vi "Main Process Case.vi"(8 "error in (no error)":errorcluster, 10 "CurrentAction":string, 11 "MPC_Laser Marked in":refnum<class "MPC_Laser Marked.lvclass">) -> (0 "error out":errorcluster, 1 "keepCase":bool, 3 "MPC_Laser Marked out":refnum<class "MPC_Laser Marked.lvclass">)   [LabVIEW 2019, in "MPC_Laser Marked.lvclass"]
uses:
  MPC_Laser Marked.lvclass
  Function/IO Folder/IO_VI/IOCtrl/Ctrl/DMC1000B_1 SelectIn.ctl
  Function/IO Folder/IO_VI/IOCtrl/Ctrl/DMC1000B_1 SelectOutput.ctl
  Function/Main UI/Ctrl/XY Table Action.ctl
  Function/UpVision/Ctrl/UpColorImg.ctl
  Function/UpVision/Ctrl/UpEnum_VisionCalibSet_Act.ctl
  Function/UpVision/Ctrl/UpGrayImg.ctl
  Function/Axis/Axis_Class/SubVI/Axis Motion/Axis_Go Point.vi
  Function/Main UI/Glb/Main_UI Gb.vi
  LLB/Commonly VI/Main Glb.vi
  LLB/Commonly VI.lvlib
  LLB/Message/MsgShowAndLog.lvlib
panel:
  out "Current Index":i32
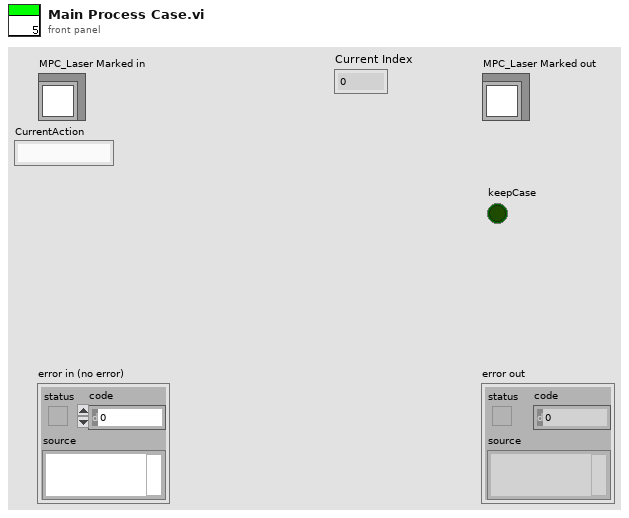
[diagram p1: front panel]
types:
  T1 = cluster{"AutoRunFlg":refnum<vi>, "Action Finish Flg":refnum<vi>, "Remaining Action":refnum<vi>, "Btn_AutoRun":refnum<vi>, "Manual Flg":refnum<vi>, "Sub Process Error":refnum<vi>}
  T2 = typedef "DMC1000B_1 SelectIn.ctl" = enum16{"M_IN00預備", "M_IN01緊急急停檢測", "M_IN02啟動按鈕綠色", "M_IN03正壓氣壓檢知", "M_IN04安全門感知", "M_IN05接受前機台有料#1信號", "M_IN06接受前機台有料#2信號", "M_IN07接受後機台要料#3信號", "M_IN08接受後機台要料#4信號", "M_IN09軌道載板前進料到位檢知", "M_IN10到料阻擋氣缸上位檢知(阻擋位)", "M_IN11到料阻擋氣缸下位檢知(阻擋位)", "M_IN12上頂固定載板氣缸上位檢知", "M_IN13上頂固定載板氣缸下位檢知", "M_IN14軌道載板到位減速檢知", "M_IN15軌道載板到位檢知", "M_IN16軌道載板後出料檢知", "M_IN17", "M_IN18", "M_IN19", "M_IN20", "M_IN21第一軸準備輸入信號 RDY", "M_IN22第二軸準備輸入信號 RDY", "M_IN23第三軸準備輸入信號 RDY", "M_IN24", "M_IN25第一軸ALM+(  伺服警報輸出  )", "M_IN26第二軸ALM+(  伺服警報輸出  )", "M_IN27第三軸ALM+(  伺服警報輸出  )", "M_IN28", "M_IN29第一軸定位完成信號 INP", "M_IN30第二軸定位完成信號 INP", "M_IN31第三軸定位完成信號 INP", "M_IN32"}
  T3 = typedef "DMC1000B_1 SelectOutput.ctl" = enum16{"M_Out0預備", "M_OUT01蜂鳴器", "M_OUT02紅燈", "M_OUT03綠燈", "M_OUT04黃燈", "M_OUT05上頂固定位氣缸電磁閥", "M_OUT06到料阻擋氣缸電磁閥", "M_OUT07向前機台發出要料#1信號", "M_OUT08向前機台發出要料#2信號", "M_OUT09向後機台發出有料#3信號", "M_OUT10向後機台發出有料#4信號", "M_OUT11接駁台馬達啟動開/關", "M_OUT12接駁台馬達慢速", "M_OUT13抽風機開/關", "M_OUT14上視覺上光源", "M_OUT15DC吹風扇開/關", "M_OUT16Z軸煞車釋放", "M_OUT17", "M_OUT18", "M_OUT19", "M_OUT20", "M_OUT21", "M_OUT22", "M_OUT23", "M_OUT24", "M_OUT25第一軸SEVON1伺服使能信號", "M_OUT26第二軸SEVON2伺服使能信號", "M_OUT27第三軸SEVON3伺服使能信號"}
  T4 = typedef "XY Table Action.ctl" = enum16{"Check Mark", "Check Z", "Laser", "Request Action"}
  T5 = enum16{"Initial", "Load", "Save", "Read", "WriteSpeed", "WritePoint"}
  T6 = cluster{"index":i32, "Mark 1Vision":cluster{"Position":cluster{"x":sgl, "y":sgl}, "Angle":sgl, "Score":sgl}, "OK/NG":bool}
  T7 = typedef "UpEnum_VisionCalibSet_Act.ctl" = enum16{"initial", "initialref", "save", "load", "UpDataToUI", "write", "read"}
  T8 = typedef "UpColorImg.ctl" = enum16{"CUpCam", "CUpSource", "CUpShow", "CUpToProcess1", "CUpToProcess2", "CUpForMatch", "CUpForCheckNumbers", "CupPreProcess"}
  T9 = typedef "UpGrayImg.ctl" = enum16{"CUpGray", "CUpProce1", "CUpProce2", "UpPattern1", "UpPattern2", "UpCalibImg", "UpPreProcess"}
  T10 = typedef "IMAQ Image.ctl" = refnum<image>
  T11 = cluster{"Position":cluster{"x":sgl, "y":sgl}, "Angle":sgl, "Score":sgl}
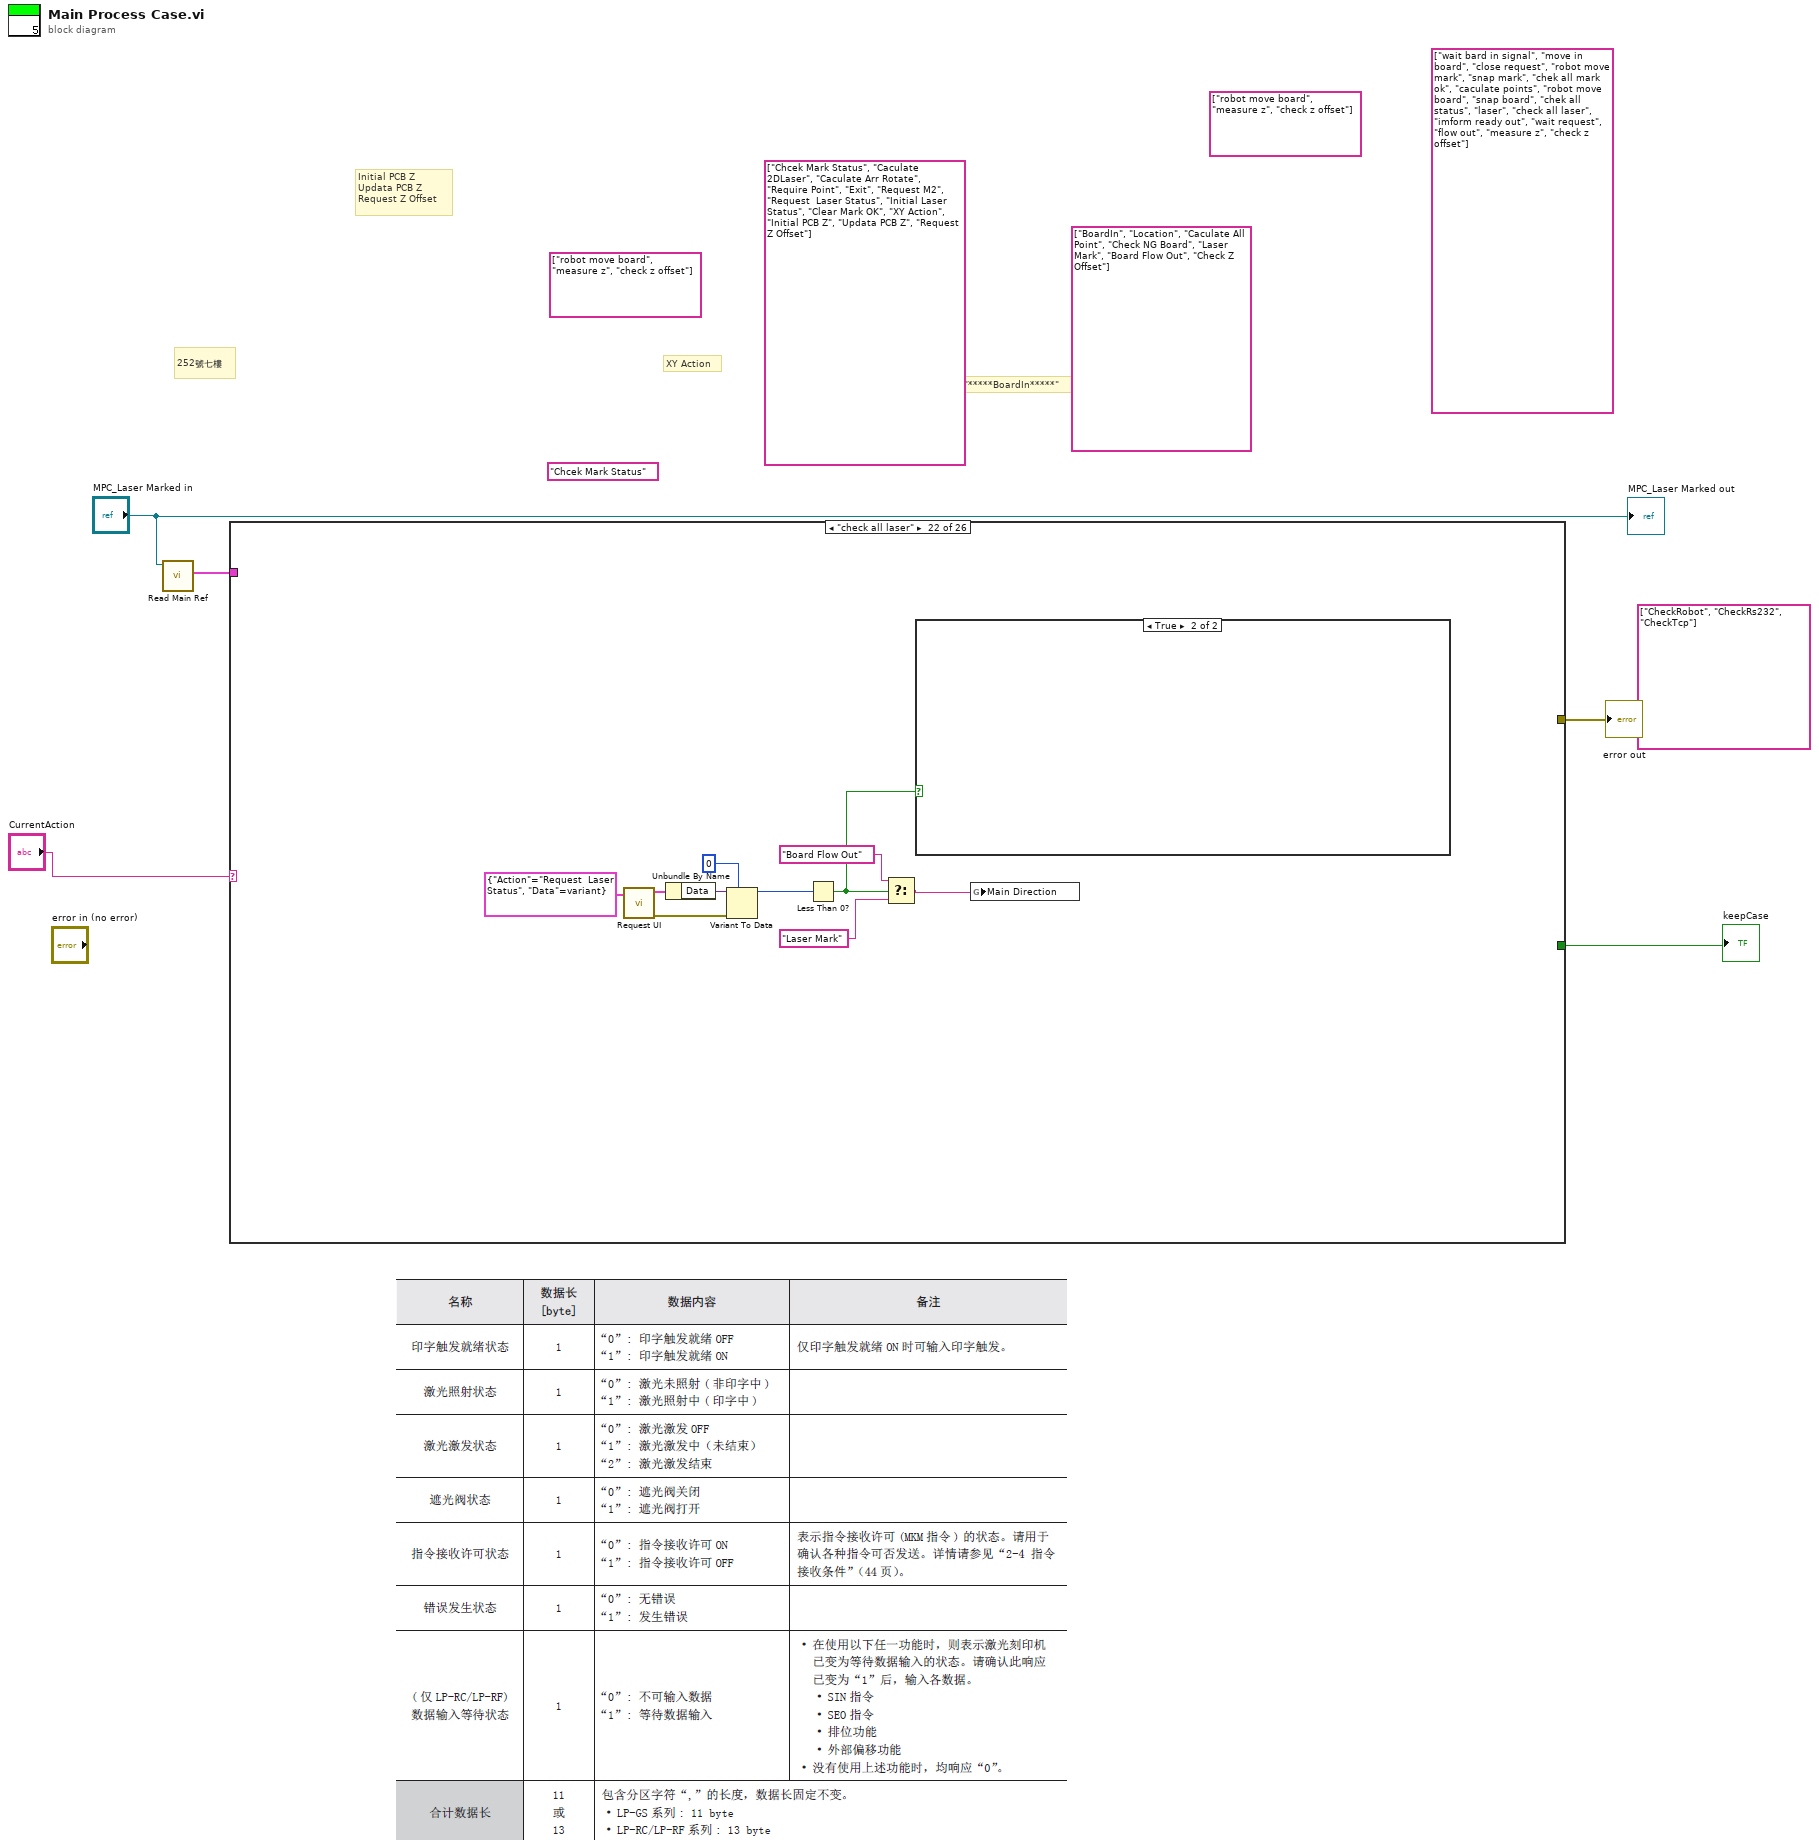
[diagram p0: block diagram]
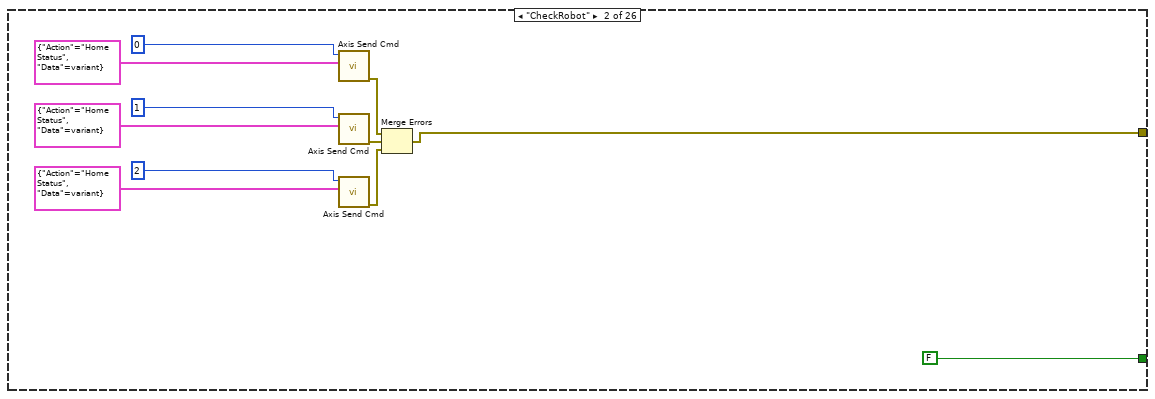
[diagram p3: hidden frame]
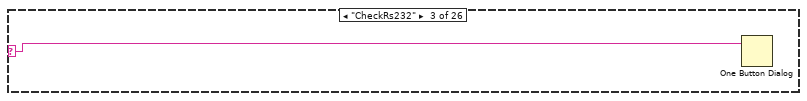
[diagram p4: hidden frame]
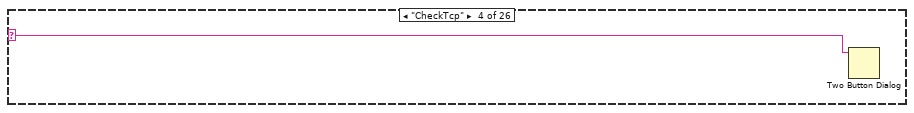
[diagram p5: hidden frame]
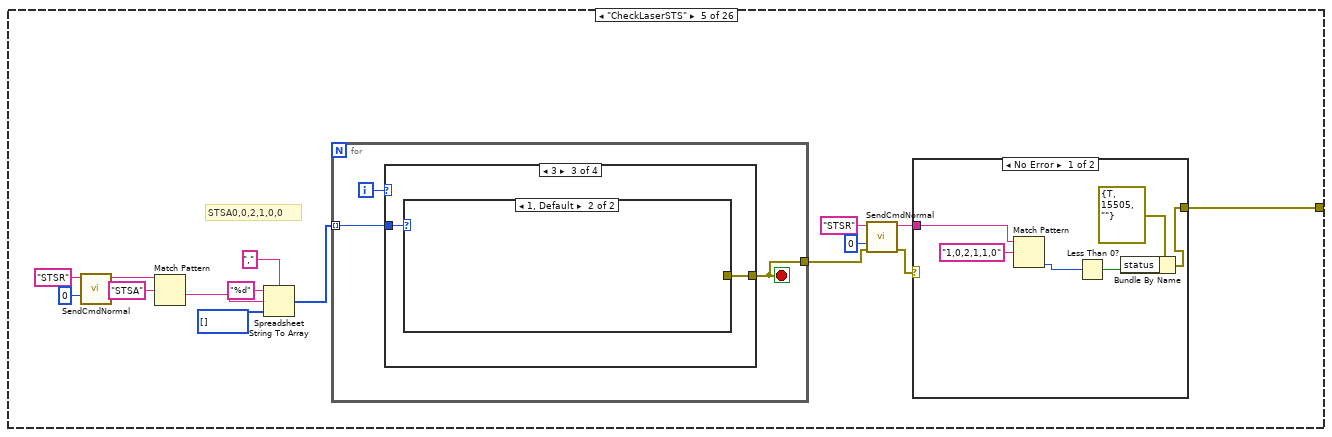
[diagram p6: hidden frame]
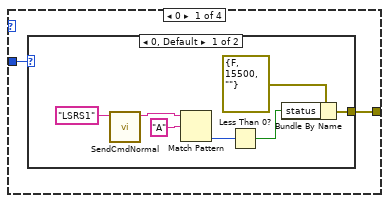
[diagram p8: hidden frame]
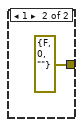
[diagram p9: hidden frame]
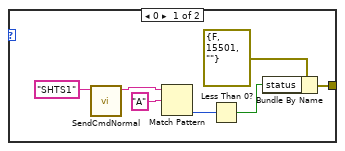
[diagram p12: hidden frame]
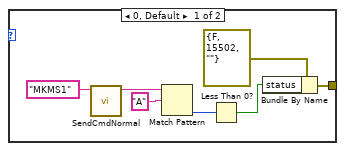
[diagram p14: hidden frame]
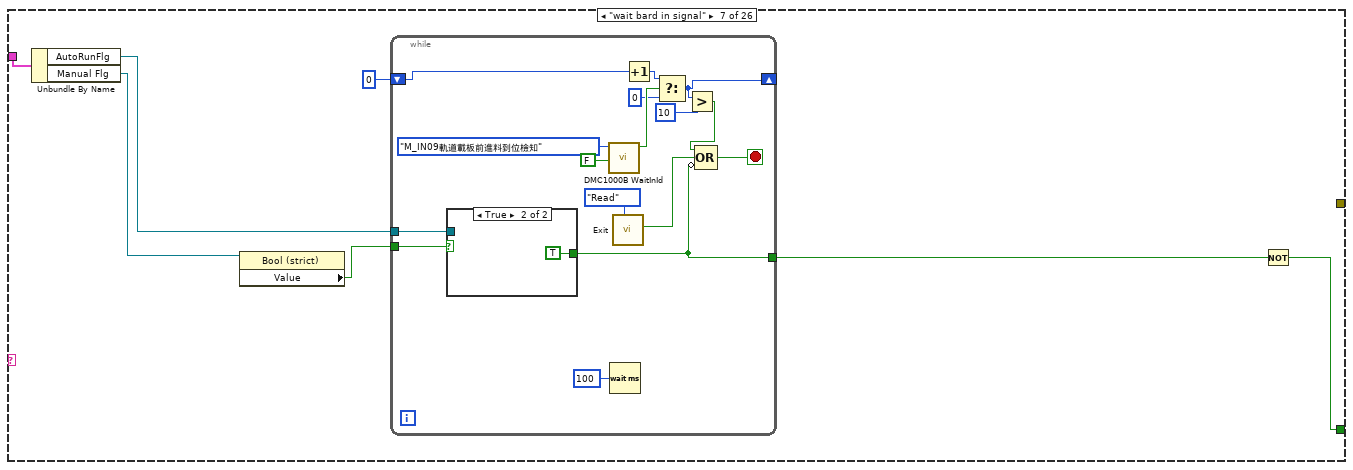
[diagram p16: hidden frame]
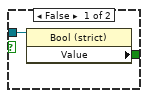
[diagram p17: hidden frame]
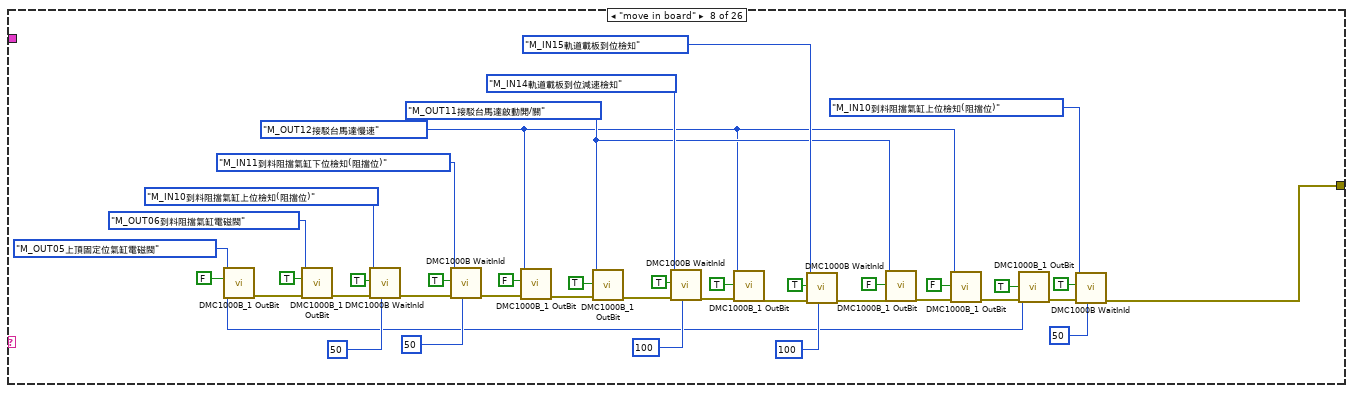
[diagram p18: hidden frame]
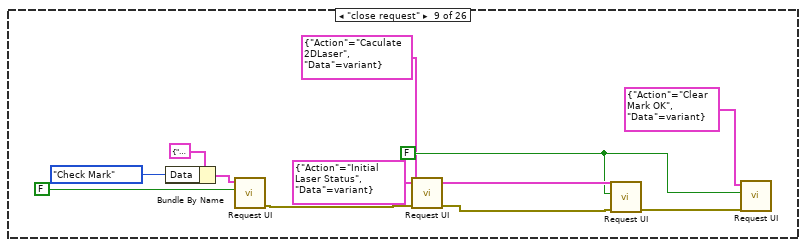
[diagram p19: hidden frame]
diagram:
  (unwired) "Chcek Mark Status" ("Action")
  (unwired) string[] ["robot move board", "measure z", "check z offset"]
  (unwired) string[] ["Chcek Mark Status", "Caculate 2DLaser", "Caculate Arr Rotate", "Require Point", "Exit", "Request M2", "Request  Laser Status", "Initial Laser Status", "Clear Mark OK", "XY Action", "Initial PCB Z", "Updata PCB Z", "Request Z Offset"]
  (unwired) string[] ["robot move board", "measure z", "check z offset"]
  (unwired) string[] ["wait bard in signal", "move in board", "close request", "robot move mark", "snap mark", "chek all mark ok", "caculate points", "robot move board", "snap board", "chek all status", "laser", "check all laser", "imform ready out", "wait request", "flow out", "measure z", "check z offset"]
  (unwired) string[] ["BoardIn", "Location", "Caculate All Point", "Check NG Board", "Laser Mark", "Board Flow Out", "Check Z Offset"]
  (unwired) string[] ["CheckRobot", "CheckRs232", "CheckTcp"] ("Process")
  # "252號七樓"
  # "Initial PCB Z\nUpdata PCB Z\nRequest Z Offset"
  # "XY Action"
  # "\"*****BoardIn*****\""
  n1 = call-dynamic "Read Main Ref.vi"("Main Process Class in"="MPC_Laser Marked in") -> ("Main Ref"=w2:T1)  [unwired: 8 in, 2 out]
  n2 = case shown="\"check all laser\"" "CurrentAction" {
    selector: "CurrentAction" -> [_ _ w17 w18 _ _ _ _ _ _ _ _ _ _ _ _ _ _ _ _ _ _ _ _ _ _]
    tunnel: [_ FALSE _ _ _ _ w77 _ _ _ _ _ _ _ _ _ _ _ _ _ _ _ _ w379 _ _] -> w4
    tunnel: w2 -> [_ _ _ _ _ _ w79 _ _ _ _ _ _ _ _ _ _ _ _ _ _ _ _ w382 _ _]
    tunnel: [_ w6 _ _ w19 _ _ w99 _ _ w156 w190 _ _ _ _ w260 w325 _ _ w356 _ _ _ w403 w410] -> w1
    frame Default {
    }
    frame "CheckRobot" {
      n3 = call "Axis Send Cmd.vi"("DataIn"=cluster{"Action":string, "Data":variant} {"Action"="Home Status", "Data"=variant}, "Axis Index"=0) -> ("Error Out"=w9:errorcluster)  [unwired: 9 in]
      n4 = call "Axis Send Cmd.vi"("DataIn"=cluster{"Action":string, "Data":variant} {"Action"="Home Status", "Data"=variant}, "Axis Index"=1) -> ("Error Out"=w8:errorcluster)  [unwired: 9 in]
      n5 = call "Axis Send Cmd.vi"("DataIn"=cluster{"Action":string, "Data":variant} {"Action"="Home Status", "Data"=variant}, "Axis Index"=2) -> ("Error Out"=w7:errorcluster)  [unwired: 9 in]
      n6 = Merge Errors(w9, w8, w7) -> (w6:errorcluster)
    }
    frame "CheckRs232" {
      n7 = One Button Dialog(message=w17) -> ()  [unwired: 1 in, 1 out]
    }
    frame "CheckTcp" {
      n8 = Two Button Dialog(message=w18) -> ()  [unwired: 2 in, 1 out]
    }
    frame "CheckLaserSTS" {
      # "STSA0,0,2,1,0,0"
      n9 = call "SendCmdNormal.vi"("index"=0, "DataIn"="STSR") -> ("Reccmd"=w31:string)  [unwired: 7 in, 2 out]
      n10 = Match Pattern(string=w31, regular expression="STSA") -> (after substring=w29:string)  [unwired: 1 in, 3 out]
      n11 = Spreadsheet String To Array(delimiter (Tab)=",", format string="%d", spreadsheet string=w29, array type (2D Dbl)=i32[] []) -> (array=w25:i32[])
      n12 = for {
        tunnel: w25 -> [w43] mode=indexing
        tunnel: [w41] -> w22
        i -> [w42]
        stop <- w41 stop-if-true
        n13 = case shown="3" w42 {
          tunnel: w43 -> [w45 w54 w56 w65]
          tunnel: [w44 _ w55 w64] -> w41
          frame 0 {
            n14 = case shown="0, Default" w45 {
              tunnel: [w47 errorcluster {"status"=FALSE, "code"=0, "source"=""} ("error out")] -> w44
              frame 0, Default {
                n15 = call "SendCmdNormal.vi"("DataIn"="LSRS1") -> ("Reccmd"=w51:string)  [unwired: 8 in, 2 out]
                n16 = Match Pattern(string=w51, regular expression="A") -> (offset past match=w49:i32)  [unwired: 1 in, 3 out]
                n17 = Less Than 0?(x=w49) -> (x < 0?=w46:bool)
                n18 = Bundle By Name(cluster=errorcluster {"status"=FALSE, "code"=15500, "source"=""} ("error constant"), "status"=w46) -> (w47:errorcluster)
              }
              frame 1 {
              }
            }
          }
          frame 1, Default {
            n19 = case shown="0, Default" w54 {
              frame 0, Default {
              }
              frame 1 {
              }
            }
          }
          frame 3 {
            n20 = case shown="1, Default" w56 {
              tunnel: [w57 _] -> w55
              frame 0 {
                n21 = call "SendCmdNormal.vi"("DataIn"="SHTS1") -> ("Reccmd"=w63:string)  [unwired: 8 in, 2 out]
                n22 = Match Pattern(string=w63, regular expression="A") -> (offset past match=w62:i32)  [unwired: 1 in, 3 out]
                n23 = Less Than 0?(x=w62) -> (x < 0?=w61:bool)
                n24 = Bundle By Name(cluster=errorcluster {"status"=FALSE, "code"=15501, "source"=""} ("error constant"), "status"=w61) -> (w57:errorcluster)
              }
              frame 1, Default {
              }
            }
          }
          frame 4 {
            n25 = case shown="1" w65 {
              tunnel: [w66 _] -> w64
              frame 0, Default {
                n26 = call "SendCmdNormal.vi"("DataIn"="MKMS1") -> ("Reccmd"=w72:string)  [unwired: 8 in, 2 out]
                n27 = Match Pattern(string=w72, regular expression="A") -> (offset past match=w71:i32)  [unwired: 1 in, 3 out]
                n28 = Less Than 0?(x=w71) -> (x < 0?=w70:bool)
                n29 = Bundle By Name(cluster=errorcluster {"status"=FALSE, "code"=15502, "source"=""} ("error constant"), "status"=w70) -> (w66:errorcluster)
              }
              frame 1 {
              }
            }
          }
        }
      }
      n30 = call "SendCmdNormal.vi"("error in (no error)"=w22, "index"=0, "DataIn"="STSR") -> ("error out"=w21:errorcluster, "Reccmd"=w20:string)  [unwired: 6 in, 1 out]
      n31 = case shown="No Error" w21 {
        selector: w21 -> [_ w40]
        tunnel: w20 -> [w39 _]
        tunnel: [w34 w40] -> w19
        frame No Error {
          n32 = Match Pattern(string=w39, regular expression="1,0,2,1,1,0") -> (offset past match=w37:i32)  [unwired: 1 in, 3 out]
          n33 = Less Than 0?(x=w37) -> (x < 0?=w36:bool)
          n34 = Bundle By Name(cluster=errorcluster {"status"=TRUE, "code"=15505, "source"=""} ("error constant"), "status"=w36) -> (w34:errorcluster)
        }
        frame Error {
        }
      }
    }
    frame "*****BoardIn*****" {
    }
    frame "wait bard in signal" {
      n35 = Unbundle By Name(w79) -> ("AutoRunFlg"=w75:refnum<vi>, "Manual Flg"=w74:refnum<vi>)
      n36 = property class="Bool (strict)"(reference=w74) -> ("Value"=w73:bool)  [unwired: 1 in, 2 out]
      n37 = while {
        tunnel: w75 -> [w92]
        tunnel: [w89] -> w78
        shift-right: [w83] -> _
        shift-left: 0 -> [w85]
        tunnel: w73 -> [w80]
        stop <- w90 stop-if-true
        n38 = case shown="True" w80 {
          tunnel: w92 -> [w97 _]
          tunnel: [w96 TRUE ("Value")] -> w89
          frame False {
            n39 = property class="Bool (strict)"(reference=w97) -> ("Value"=w96:bool)  [unwired: 1 in, 2 out]
          }
          frame True {
          }
        }
        n40 = call "DMC1000B WaitInId.vi"("Wait?"=FALSE, "64IIN_4 Select"=DMC1000B_1_SelectIn."M_IN09軌道載板前進料到位檢知") -> ("StatusOut"=w87:bool)  [unwired: 7 in, 2 out]
        n41 = Wait (ms)(milliseconds to wait=u32 100) -> ()  [unwired: 1 out]
        n42 = call "Exit.vi"("Enum"=enum16{"Initial", "Read", "Write"}."Read") -> ("ExitOut"=w91:bool)  [unwired: 10 in]
        n43 = Increment(x=w85) -> (x+1=w86:i32)
        n44 = Select(t=w86, s=w87, f=0) -> (s? t:f=w83:i32)
        n45 = Greater?(x=w83, y=10) -> (0:w81:bool)
        n46 = Compound Arithmetic op=OR(w81, w91, invert w89) -> (w90:bool)
      }
      n47 = Not(x=w78) -> (.not. x?=w77:bool)
    }
    frame "move in board" {
      w107 = DMC1000B_1_SelectOutput."M_OUT12接駁台馬達慢速" ("IO_Output_1 Select")
      w110 = DMC1000B_1_SelectOutput."M_OUT11接駁台馬達啟動開/關" ("IO_Output_1 Select")
      w104 = DMC1000B_1_SelectOutput."M_OUT05上頂固定位氣缸電磁閥" ("IO_Output_1 Select")
      n48 = call "DMC1000B_1 OutBit.vi"("BL"=FALSE, "IO_Output_1 Select"=w104) -> ("error out"=w128:errorcluster)  [unwired: 9 in]
      n49 = call "DMC1000B_1 OutBit.vi"("error in (no error)"=w128, "BL"=TRUE, "IO_Output_1 Select"=DMC1000B_1_SelectOutput."M_OUT06到料阻擋氣缸電磁閥") -> ("error out"=w133:errorcluster)  [unwired: 8 in]
      n50 = call "DMC1000B WaitInId.vi"("time(0.1)"=50, "error in"=w133, "Status"=TRUE, "64IIN_4 Select"=DMC1000B_1_SelectIn."M_IN10到料阻擋氣缸上位檢知(阻擋位)") -> ("error Out"=w127:errorcluster)  [unwired: 5 in, 2 out]
      n51 = call "DMC1000B WaitInId.vi"("time(0.1)"=50, "error in"=w127, "Status"=TRUE, "64IIN_4 Select"=DMC1000B_1_SelectIn."M_IN11到料阻擋氣缸下位檢知(阻擋位)") -> ("error Out"=w116:errorcluster)  [unwired: 5 in, 2 out]
      n52 = call "DMC1000B_1 OutBit.vi"("error in (no error)"=w116, "BL"=FALSE, "IO_Output_1 Select"=w107) -> ("error out"=w115:errorcluster)  [unwired: 8 in]
      n53 = call "DMC1000B_1 OutBit.vi"("error in (no error)"=w115, "BL"=TRUE, "IO_Output_1 Select"=w110) -> ("error out"=w124:errorcluster)  [unwired: 8 in]
      n54 = call "DMC1000B WaitInId.vi"("time(0.1)"=100, "error in"=w124, "Status"=TRUE, "64IIN_4 Select"=DMC1000B_1_SelectIn."M_IN14軌道載板到位減速檢知") -> ("error Out"=w118:errorcluster)  [unwired: 5 in, 2 out]
      n55 = call "DMC1000B_1 OutBit.vi"("error in (no error)"=w118, "BL"=TRUE, "IO_Output_1 Select"=w107) -> ("error out"=w117:errorcluster)  [unwired: 8 in]
      n56 = call "DMC1000B WaitInId.vi"("time(0.1)"=100, "error in"=w117, "Status"=TRUE, "64IIN_4 Select"=DMC1000B_1_SelectIn."M_IN15軌道載板到位檢知") -> ("error Out"=w111:errorcluster)  [unwired: 5 in, 2 out]
      n57 = call "DMC1000B_1 OutBit.vi"("error in (no error)"=w111, "BL"=FALSE, "IO_Output_1 Select"=w110) -> ("error out"=w108:errorcluster)  [unwired: 8 in]
      n58 = call "DMC1000B_1 OutBit.vi"("error in (no error)"=w108, "BL"=FALSE, "IO_Output_1 Select"=w107) -> ("error out"=w105:errorcluster)  [unwired: 8 in]
      n59 = call "DMC1000B_1 OutBit.vi"("error in (no error)"=w105, "BL"=TRUE, "IO_Output_1 Select"=w104) -> ("error out"=w103:errorcluster)  [unwired: 8 in]
      n60 = call "DMC1000B WaitInId.vi"("time(0.1)"=50, "error in"=w103, "Status"=TRUE, "64IIN_4 Select"=DMC1000B_1_SelectIn."M_IN10到料阻擋氣缸上位檢知(阻擋位)") -> ("error Out"=w99:errorcluster)  [unwired: 5 in, 2 out]
    }
    frame "close request" {
      w146 = FALSE ("Wait Reply")
      n61 = Bundle By Name(cluster=cluster{"Action":string, "Data":variant} {"Action"="XY Action", "Data"=variant} ("Data"), "Data"=XY_Table_Action."Check Mark" ("XY Table Action")) -> (w143:cluster{"Action":string, "Data":variant})
      n62 = call "Request UI.vi"("Wait Reply"=FALSE, "Data"=w143) -> ("error out"=w141:errorcluster)  [unwired: 8 in, 1 out]
      n63 = call "Request UI.vi"("error in (no error)"=w141, "Data"=cluster{"Action":string, "Data":variant} {"Action"="Caculate 2DLaser", "Data"=variant}) -> ("error out"=w144:errorcluster)  [unwired: 8 in, 1 out]
      n64 = call "Request UI.vi"("error in (no error)"=w144, "Wait Reply"=w146, "Data"=cluster{"Action":string, "Data":variant} {"Action"="Initial Laser Status", "Data"=variant}) -> ("error out"=w147:errorcluster)  [unwired: 7 in, 1 out]
      n65 = call "Request UI.vi"("error in (no error)"=w147, "Wait Reply"=w146, "Data"=cluster{"Action":string, "Data":variant} {"Action"="Clear Mark OK", "Data"=variant}) -> ()  [unwired: 7 in, 2 out]
    }
    frame "*****Location*****" {
    }
    frame "robot move mark" {
      n66 = call "Request UI.vi"("Data"=cluster{"Action":string, "Data":variant} {"Action"="Chcek Mark Status", "Data"=variant}) -> ("DataOut"=w154:cluster{"Action":string, "Data":variant})  [unwired: 9 in, 1 out]
      n67 = Unbundle By Name(w154) -> ("Data"=w153:variant)
      n68 = Variant To Data(type=cluster{"M1":bool, "M2":bool} {"M1"=TRUE, "M2"=TRUE}, Variant=w153) -> (data=w151:cluster{"M1":bool, "M2":bool})  [unwired: 1 in, 1 out]
      n69 = Unbundle(w151) -> ("M1"=w150:bool)  [unwired: 1 out]
      n70 = case shown="True" w150 {
        tunnel: [w158 w164] -> w157
        frame False {
          n71 = call "Axis_Point Table.vi"("Enum"=T5."Read") -> ("RobotPoint"=w162:string[][])  [unwired: 8 in, 2 out]
          n72 = call "SelectPoint.vi"("PointName"="Mark1", "RobotPointsTableIn"=w162) -> ("RobotPointsOut"=w160:string[][])  [unwired: 7 in, 2 out]
          n73 = Index Array(array=w160, index (row)=0) -> (element=w158:string[])  [unwired: 1 in]
        }
        frame True {
          w167 = 2 ("index")
          w168 = 1 ("index")
          n74 = call "Axis_Point Table.vi"("Enum"=T5."Read") -> ("RobotPoint"=w186:string[][])  [unwired: 8 in, 2 out]
          n75 = call "Request UI.vi"("Data"=cluster{"Action":string, "Data":variant} {"Action"="Request M2", "Data"=variant}) -> ("DataOut"=w179:cluster{"Action":string, "Data":variant})  [unwired: 9 in, 1 out]
          n76 = Unbundle By Name(w179) -> ("Data"=w180:variant)
          n77 = call "SelectPoint.vi"("PointName"="Mark1", "RobotPointsTableIn"=w186) -> ("RobotPointsOut"=w185:string[][])  [unwired: 7 in, 2 out]
          n78 = Variant To Data(type=cluster{"X":dbl, "Y":dbl} {"X"=100.0, "Y"=50.0} ("Mark 2"), Variant=w180) -> (data=w176:cluster{"X":dbl, "Y":dbl})  [unwired: 1 in, 1 out]
          n79 = Index Array(array=w185, index (row)=0) -> (element=w169:string[])  [unwired: 1 in]
          n80 = Fract/Exp String To Number(string=w169) -> (number=w177:dbl[])  [unwired: 3 in, 1 out]
          n81 = Unbundle(w176) -> ("X"=w174:dbl, "Y"=w172:dbl)
          n82 = Index Array(array=w177, index #1=w168, index #2=w167) -> (element #1=w175:dbl, element #2=w173:dbl)
          n83 = Add(x=w175, y=w174) -> (x+y=w171:dbl)
          n84 = Add(x=w173, y=w172) -> (x+y=w170:dbl)
          n85 = Number To Fractional String(number=w171) -> (F-format string=w166:string)  [unwired: 3 in]
          n86 = Number To Fractional String(number=w170) -> (F-format string=w165:string)  [unwired: 3 in]
          n87 = Replace Array Subset(array=w169, new element #1=w166, index #1=w168, new element #2=w165, index #2=w167) -> (w164:string[])
        }
      }
      n88 = call-poly "Axis Motion.vi"("RobotPoints in"=w157) -> ("error out"=w156:errorcluster)  [unwired: 10 in]
    }
    frame "snap mark" {
      # "Update Mark Data"
      n89 = global read "Main_UI Gb.vi" "Image Glb"() -> (w189:variant)
      n90 = Variant To Data(type=refnum<vi> refnum ("Image"), Variant=w189) -> (data=w187:refnum<vi>)  [unwired: 1 in, 1 out]
      n91 = call "DMC1000B_1 OutBit.vi"("BL"=TRUE, "IO_Output_1 Select"=DMC1000B_1_SelectOutput."M_OUT14上視覺上光源") -> ("error out"=w193:errorcluster)  [unwired: 9 in]
      n92 = for {
        N: 2 -> [_]
        tunnel: [w205] -> w190
        tunnel: cluster{"Action":string, "Data":variant} {"Action"="Chcek Mark Status", "Data"=variant} ("Data") -> [w200]
        tunnel: w193 -> [_]
        tunnel: w187 -> [w199]
        stop <- w203 stop-if-true
        n93 = call "Request UI.vi"("Data"=w200) -> ("DataOut"=w221:cluster{"Action":string, "Data":variant})  [unwired: 9 in, 1 out]
        n94 = Unbundle By Name(w221) -> ("Data"=w220:variant)
        n95 = call "Wait t.vi"("wait(ms)"=u32 500) -> ("error out"=w225:errorcluster)  [unwired: 10 in]
        n96 = call "UpImgCtrl.vi"("Action"=enum16{"Initial", "read", "release"}."read", "error in (no error)"=w225, "ColorImg 2"=UpColorImg."CUpSource") -> ("error out"=w224:errorcluster, "ColorImg"=w227:string)  [unwired: 6 in, 1 out]
        n97 = call "UpImgCtrl.vi"("Action"=enum16{"Initial", "read", "release"}."read", "ColorImg 2"=UpColorImg."CUpToProcess1") -> ("ColorImg"=w226:string)  [unwired: 7 in, 2 out]
        n98 = Variant To Data(type=cluster{"M1":bool, "M2":bool} {"M1"=TRUE, "M2"=TRUE}, Variant=w220) -> (data=w219:cluster{"M1":bool, "M2":bool})  [unwired: 1 in, 1 out]
        n99 = call "IMAQ Copy"("error in (no error)"=w224, "Image Dst"=w226, "Image Src"=w227) -> ("Image Dst Out"=w223:T10)  [unwired: 3 in, 1 out]
        n100 = Unbundle(w219) -> ("M1"=w217:bool)  [unwired: 1 out]
        n101 = case shown="True" w217 {
          tunnel: [cluster{"Y":i32, "X":i32} {"Y"=1, "X"=0} ("indedx") cluster{"Y":i32, "X":i32} {"Y"=1, "X"=1} ("indedx")] -> w216
          tunnel: [UpGrayImg."UpPattern1" ("GrayImg 2") UpGrayImg."UpPattern2" ("GrayImg 2")] -> w213
          tunnel: [0 1] -> w209
          frame False {
          }
          frame True {
          }
        }
        n102 = call "UpVisionAlgSet.vi"("Enum"=UpEnum_VisionCalibSet_Act."read", "indedx"=w216) -> ("DataOut"=w215:string)  [unwired: 7 in, 2 out]
        n103 = call "UpImgCtrl.vi"("Action"=enum16{"Initial", "read", "release"}."read", "GrayImg 2"=w213) -> ("GrayImg"=w212:string)  [unwired: 7 in, 2 out]
        n104 = call "Up_PatternMatch.vi"("Image In"=w223, "Template Image"=w212, "ROIIn"=w215) -> ("Image Out"=w198:T10, "ResultShow"=w208:T11, "OK"=w203:bool)  [unwired: 6 in, 4 out]
        n105 = disable-structure shown="Disabled" {
          disable-tunnel: w199 -> [w234 _]
          disable-tunnel: w198 -> [w233 _]
          frame Disabled {
            n106 = property class="ImageControl"(reference=w234, "Value"=w233) -> ()  [unwired: 1 in, 2 out]
          }
          frame Enabled {
          }
        }
        n107 = Bundle(cluster=T6 {"index"=0, "Mark 1Vision"={"Position"={"x"=0.0, "y"=0.0}, "Angle"=0.0, "Score"=0.0}, "OK/NG"=FALSE}, "index"=w209, "Mark 1Vision"=w208, "OK/NG"=w203) -> (w207:T6)
        n108 = Bundle By Name(cluster=cluster{"Action":string, "Data":variant} {"Action"="Update Mark Data", "Data"=variant} ("Data"), "Data"=w207) -> (w206:cluster{"Action":string, "Data":variant})
        n109 = Not(x=w203) -> (.not. x?=w202:bool)
        n110 = call "Request UI.vi"("Data"=w206) -> ()  [unwired: 9 in, 2 out]
        n111 = Bundle By Name(cluster=errorcluster {"status"=FALSE, "code"=0, "source"=""} ("error constant"), "status"=w202, "code"=10102) -> (w205:errorcluster)
      }
      n112 = call "DMC1000B_1 OutBit.vi"("error in (no error)"=w190, "BL"=FALSE, "IO_Output_1 Select"=DMC1000B_1_SelectOutput."M_OUT14上視覺上光源") -> ()  [unwired: 8 in, 1 out]
    }
    frame "chek all mark ok" {
      n113 = Bundle By Name(cluster=cluster{"Action":string, "Data":variant} {"Action"="Chcek Mark Status", "Data"=variant} ("Data"), "Action"="Chcek Mark Status") -> (w242:cluster{"Action":string, "Data":variant})
      n114 = call "Request UI.vi"("Data"=w242) -> ("DataOut"=w253:cluster{"Action":string, "Data":variant})  [unwired: 9 in, 1 out]
      n115 = Unbundle By Name(w253) -> ("Data"=w252:variant)
      n116 = Variant To Data(type=cluster{"M1":bool, "M2":bool} {"M1"=TRUE, "M2"=TRUE}, Variant=w252) -> (data=w251:cluster{"M1":bool, "M2":bool})  [unwired: 1 in, 1 out]
      n117 = Unbundle(w251) -> ("M1"=w249:bool, "M2"=w248:bool)
      n118 = And(x=w249, y=w248) -> (x .and. y?=w247:bool)
      n119 = Select(t="Caculate All Point", s=w247, f="Location") -> (s? t:f=w246:string)
      n120 = global write "Main Glb.vi" "Main Direction"(w246) -> ()
    }
    frame "*****Caculate All Point*****" {
    }
    frame "caculate points" {
      n121 = call "Request UI.vi"("Data"=cluster{"Action":string, "Data":variant} {"Action"="Caculate Arr Rotate", "Data"=variant}) -> ("error out"=w254:errorcluster)  [unwired: 9 in, 1 out]
      n122 = Bundle By Name(cluster=cluster{"Action":string, "Data":variant} {"Action"="XY Action", "Data"=variant} ("Data"), "Data"=XY_Table_Action."Check Z" ("XY Table Action")) -> (w258:cluster{"Action":string, "Data":variant})
      n123 = call "Request UI.vi"("error in (no error)"=w254, "Wait Reply"=FALSE, "Data"=w258) -> ()  [unwired: 7 in, 2 out]
    }
    frame "*****Check Z Offset*****" {
    }
    frame "robot move board" {
      w262 = XY_Table_Action."Request Action" ("XY Table Action")
      n124 = Bundle By Name(cluster=cluster{"Action":string, "Data":variant} {"Action"="XY Action", "Data"=variant} ("Data"), "Data"=w262) -> (w264:cluster{"Action":string, "Data":variant})
      n125 = call "Request UI.vi"("Data"=w264) -> ("DataOut"=w265:cluster{"Action":string, "Data":variant})  [unwired: 9 in, 1 out]
      n126 = Unbundle By Name(w265) -> ("Data"=w266:variant)
      n127 = Variant To Data(type=w262, Variant=w266) -> (data=w263:T4)  [unwired: 1 in, 1 out]
      n128 = case shown="\"Laser\"" w263 {
        tunnel: [w277 w309] -> w267
        frame "Check Z", Default {
          w284 = 0.0
          n129 = call "Request UI.vi"("Data"=cluster{"Action":string, "Data":variant} {"Action"="Request  Laser Status", "Data"=variant}) -> ("error out"=w296:errorcluster, "DataOut"=w292:cluster{"Action":string, "Data":variant})  [unwired: 9 in]
          n130 = call "SystemSearchDataName.vi"("element"="$Laser Tool Y") -> ("variant"=w285:variant)  [unwired: 8 in, 2 out]
          n131 = Unbundle By Name(w292) -> ("Data"=w293:variant)
          n132 = call "SystemSearchDataName.vi"("element"="$Laser Tool X") -> ("variant"=w286:variant)  [unwired: 8 in, 2 out]
          n133 = Variant To Data(type=w284, Variant=w285) -> (data=w279:dbl)  [unwired: 1 in, 1 out]
          n134 = Variant To Data(type=w284, Variant=w286) -> (data=w281:dbl)  [unwired: 1 in, 1 out]
          n135 = Variant To Data(error in=w296, type=0, Variant=w293) -> (data=w268:i32, error out=w297:errorcluster)
          "Current Index" <- w268
          n136 = Bundle By Name(cluster=cluster{"Action":string, "Data":variant} {"Action"="Require Point", "Data"=variant} ("Data"), "Data"=w268) -> (w269:cluster{"Action":string, "Data":variant})
          n137 = call "Request UI.vi"("error in (no error)"=w297, "Data"=w269) -> ("error out"=w298:errorcluster, "DataOut"=w295:cluster{"Action":string, "Data":variant})  [unwired: 8 in]
          n138 = Unbundle By Name(w295) -> ("Data"=w294:variant)
          n139 = Variant To Data(error in=w298, type=cluster{"X":dbl, "Y":dbl, "Angle":dbl} {"X"=0.0, "Y"=0.0, "Angle"=0.0} ("element"), Variant=w294) -> (data=w283:cluster{"X":dbl, "Y":dbl, "Angle":dbl})  [unwired: 1 out]
          n140 = Unbundle(w283) -> ("X"=w282:dbl, "Y"=w280:dbl)  [unwired: 1 out]
          n141 = Add(x=w280, y=w279) -> (x+y=w275:dbl)
          n142 = Add(x=w282, y=w281) -> (x+y=w276:dbl)
          n143 = Number To Fractional String(number=w276) -> (F-format string=w272:string)  [unwired: 3 in]
          n144 = Number To Fractional String(number=w275) -> (F-format string=w271:string)  [unwired: 3 in]
          n145 = Replace Array Subset(array=string[] ["Name", "X", "Y", "Z"] ("RobotPointsOut"), new element #1=w272, index #1=1 ("index"), new element #2=w271, index #2=2 ("index")) -> (w277:string[])
        }
        frame "Laser" {
          w299 = 0.0
          n146 = call "Request UI.vi"("Data"=cluster{"Action":string, "Data":variant} {"Action"="Request  Laser Status", "Data"=variant}) -> ("error out"=w321:errorcluster, "DataOut"=w317:cluster{"Action":string, "Data":variant})  [unwired: 9 in]
          n147 = Unbundle By Name(w317) -> ("Data"=w318:variant)
          n148 = Variant To Data(error in=w321, type=0, Variant=w318) -> (data=w300:i32, error out=w322:errorcluster)
          n149 = Bundle By Name(cluster=cluster{"Action":string, "Data":variant} {"Action"="Require Point", "Data"=variant} ("Data"), "Data"=w300) -> (w301:cluster{"Action":string, "Data":variant})
          n150 = local write "Current Index"(w300) -> ()
          n151 = call "Request UI.vi"("error in (no error)"=w322, "Data"=w301) -> ("error out"=w323:errorcluster, "DataOut"=w320:cluster{"Action":string, "Data":variant})  [unwired: 8 in]
          n152 = Unbundle By Name(w320) -> ("Data"=w319:variant)
          n153 = Variant To Data(error in=w323, type=cluster{"X":dbl, "Y":dbl, "Angle":dbl} {"X"=0.0, "Y"=0.0, "Angle"=0.0} ("element"), Variant=w319) -> (data=w313:cluster{"X":dbl, "Y":dbl, "Angle":dbl})  [unwired: 1 out]
          n154 = Unbundle(w313) -> ("X"=w312:dbl, "Y"=w311:dbl)  [unwired: 1 out]
          n155 = Add(x=w311, y=w299) -> (x+y=w307:dbl)
          n156 = Add(x=w312, y=w299) -> (x+y=w308:dbl)
          n157 = Number To Fractional String(number=w308) -> (F-format string=w304:string)  [unwired: 3 in]
          n158 = Number To Fractional String(number=w307) -> (F-format string=w303:string)  [unwired: 3 in]
          n159 = Replace Array Subset(array=string[] ["Name", "X", "Y", "Z"] ("RobotPointsOut"), new element #1=w304, index #1=1 ("index"), new element #2=w303, index #2=2 ("index")) -> (w309:string[])
        }
      }
      n160 = call-poly "Axis Motion.vi"("RobotPoints in"=w267) -> ("error out"=w260:errorcluster)  [unwired: 10 in]
    }
    frame "measure z" {
      n161 = call "Laser.vi"() -> ("error Out"=w324:errorcluster, "Laser1"=w326:dbl)  [unwired: 10 in]
      n162 = case shown="No Error" w324 {
        selector: w324 -> [_ w336]
        tunnel: w326 -> [w333 _]
        tunnel: [errorcluster {"status"=FALSE, "code"=0, "source"=""} ("error IO") w336] -> w325
        frame No Error {
          n163 = local read "Current Index"() -> (w328:i32)
          n164 = Bundle By Name(cluster=cluster{"Action":string, "Data":variant} {"Action"="Updata Laser Status", "Data"=variant} ("Data"), "Data"=w328) -> (w330:cluster{"Action":string, "Data":variant})
          n165 = call "Request UI.vi"("Data"=w330) -> ("error out"=w329:errorcluster)  [unwired: 9 in, 1 out]
          n166 = Bundle("Current Index"=w328, "Laser1"=w333) -> (w332:cluster{"Current Index":i32, "Laser1":dbl})  [unwired: 1 in]
          n167 = Bundle By Name(cluster=cluster{"Action":string, "Data":variant} {"Action"="Updata PCB Z", "Data"=variant} ("Data"), "Data"=w332) -> (w335:cluster{"Action":string, "Data":variant})
          n168 = call "Request UI.vi"("error in (no error)"=w329, "Data"=w335) -> ()  [unwired: 8 in, 2 out]
        }
        frame Error {
        }
      }
    }
    frame "check z offset" {
      n169 = call "Request UI.vi"("Data"=cluster{"Action":string, "Data":variant} {"Action"="Request  Laser Status", "Data"=variant}) -> ("error out"=w346:errorcluster, "DataOut"=w344:cluster{"Action":string, "Data":variant})  [unwired: 9 in]
      n170 = Unbundle By Name(w344) -> ("Data"=w345:variant)
      n171 = Variant To Data(error in=w346, type=0, Variant=w345) -> (data=w341:i32)  [unwired: 1 out]
      n172 = Less Than 0?(x=w341) -> (x < 0?=w337:bool)
      n173 = Select(t="Laser Mark", s=w337, f="Check Z Offset") -> (s? t:f=w338:string)
      n174 = case shown="True" w337 {
        frame False {
        }
        frame True {
          n175 = call "Request UI.vi"("Wait Reply"=FALSE, "Data"=cluster{"Action":string, "Data":variant} {"Action"="Initial Laser Status", "Data"=variant}) -> ("error out"=w353:errorcluster)  [unwired: 8 in, 1 out]
          n176 = Bundle By Name(cluster=cluster{"Action":string, "Data":variant} {"Action"="XY Action", "Data"=variant} ("Data"), "Data"=XY_Table_Action."Laser" ("XY Table Action")) -> (w352:cluster{"Action":string, "Data":variant})
          n177 = call "Request UI.vi"("error in (no error)"=w353, "Wait Reply"=FALSE, "Data"=w352) -> ()  [unwired: 7 in, 2 out]
        }
      }
      n178 = global write "Main Glb.vi" "Main Direction"(w338) -> ()
    }
    frame "*****Laser Mark*****" {
    }
    frame "laser" {
      n179 = call "Request UI.vi"("Data"=cluster{"Action":string, "Data":variant} {"Action"="Request SN", "Data"=variant}) -> ("DataOut"=w360:cluster{"Action":string, "Data":variant})  [unwired: 9 in, 1 out]
      n180 = Unbundle By Name(w360) -> ("Data"=w359:variant)
      n181 = Variant To Data(type="", Variant=w359) -> (data=w354:string)  [unwired: 1 in, 1 out]
      n182 = call "Laser MARKED V1.vi"("Sn"=w354, "Marked Type"="bf1-1") -> ("error constant"=w357:errorcluster)  [unwired: 9 in]
      n183 = case shown="No Error" w357 {
        selector: w357 -> [_ w366]
        tunnel: [w362 w366] -> w356
        frame No Error {
          n184 = local read "Current Index"() -> (w364:i32)
          n185 = Bundle By Name(cluster=cluster{"Action":string, "Data":variant} {"Action"="Updata Laser Status", "Data"=variant} ("Data"), "Data"=w364) -> (w365:cluster{"Action":string, "Data":variant})
          n186 = call "Request UI.vi"("Data"=w365) -> ("error out"=w362:errorcluster)  [unwired: 9 in, 1 out]
        }
        frame Error {
        }
      }
    }
    frame "check all laser" {
      n187 = call "Request UI.vi"("Data"=cluster{"Action":string, "Data":variant} {"Action"="Request  Laser Status", "Data"=variant}) -> ("error out"=w376:errorcluster, "DataOut"=w374:cluster{"Action":string, "Data":variant})  [unwired: 9 in]
      n188 = Unbundle By Name(w374) -> ("Data"=w375:variant)
      n189 = Variant To Data(error in=w376, type=0, Variant=w375) -> (data=w373:i32)  [unwired: 1 out]
      n190 = Less Than 0?(x=w373) -> (x < 0?=w371:bool)
      n191 = Select(t="Board Flow Out", s=w371, f="Laser Mark") -> (s? t:f=w372:string)
      n192 = case shown="True" w371 {
        frame False {
        }
        frame True {
        }
      }
      n193 = global write "Main Glb.vi" "Main Direction"(w372) -> ()
    }
    frame "*****Board Flow Out*****" {
    }
    frame "imform ready out" {
      n194 = Unbundle By Name(w382) -> ("AutoRunFlg"=w381:refnum<vi>, "Manual Flg"=w378:refnum<vi>)
      n195 = property class="Bool (strict)"(reference=w378) -> ("Value"=w377:bool)  [unwired: 1 in, 2 out]
      n196 = while {
        tunnel: w381 -> [w396]
        tunnel: [w393] -> w380
        shift-right: [w389] -> _
        shift-left: 0 -> [w390]
        tunnel: w377 -> [w384]
        stop <- w394 stop-if-true
        n197 = case shown="True" w384 {
          tunnel: w396 -> [w401 _]
          tunnel: [w400 TRUE ("Value")] -> w393
          frame False {
            n198 = property class="Bool (strict)"(reference=w401) -> ("Value"=w400:bool)  [unwired: 1 in, 2 out]
          }
          frame True {
          }
        }
        n199 = Wait (ms)(milliseconds to wait=u32 100) -> ()  [unwired: 1 out]
        n200 = call "DMC1000B WaitInId.vi"("Wait?"=FALSE, "64IIN_4 Select"=DMC1000B_1_SelectIn."M_IN16軌道載板後出料檢知") -> ("StatusOut"=w391:bool)  [unwired: 7 in, 2 out]
        n201 = call "Exit.vi"("Enum"=enum16{"Initial", "Read", "Write"}."Read") -> ("ExitOut"=w395:bool)  [unwired: 10 in]
        n202 = Increment(x=w390) -> (x+1=w386:i32)
        n203 = Select(t=0 ("f"), s=w391, f=w386) -> (s? t:f=w389:i32)
        n204 = Greater?(x=w389, y=5) -> (0:w387:bool)
        n205 = Compound Arithmetic op=OR(w387, w395, invert w393) -> (w394:bool)
      }
      n206 = Not(x=w380) -> (.not. x?=w379:bool)
    }
    frame "wait request" {
      n207 = call "DMC1000B_1 OutBit.vi"("BL"=FALSE, "IO_Output_1 Select"=DMC1000B_1_SelectOutput."M_OUT05上頂固定位氣缸電磁閥") -> ("error out"=w404:errorcluster)  [unwired: 9 in]
      n208 = call "DMC1000B WaitInId.vi"("time(0.1)"=50, "error in"=w404, "Status"=TRUE, "64IIN_4 Select"=DMC1000B_1_SelectIn."M_IN11到料阻擋氣缸下位檢知(阻擋位)") -> ("error Out"=w403:errorcluster)  [unwired: 5 in, 2 out]
    }
    frame "flow out" {
      n209 = call "DMC1000B_1 OutBit.vi"("BL"=TRUE, "IO_Output_1 Select"=DMC1000B_1_SelectOutput."M_OUT11接駁台馬達啟動開/關") -> ("error out"=w411:errorcluster)  [unwired: 9 in]
      n210 = call "DMC1000B WaitInId.vi"("time(0.1)"=50, "error in"=w411, "Status"=TRUE, "64IIN_4 Select"=DMC1000B_1_SelectIn."M_IN16軌道載板後出料檢知") -> ("error Out"=w410:errorcluster)  [unwired: 5 in, 2 out]
      n211 = flat-sequence {
        tunnel: w410 -> [_]
        frame #0 {
          n212 = call "DMC1000B_1 OutBit.vi"("BL"=FALSE, "IO_Output_1 Select"=DMC1000B_1_SelectOutput."M_OUT11接駁台馬達啟動開/關") -> ()  [unwired: 9 in, 1 out]
        }
      }
    }
  }
  "error out" <- w1
  "keepCase" <- w4
  "MPC_Laser Marked out" <- "MPC_Laser Marked in"
